vi "Act_cmd (SubVI).vi"(4 "W_b [rad/s]":dbl[](array[numeric]), 6 "Angles [rad]":dbl[](array[numeric]), 8 "TVA_old [rad]":dbl[](array[numeric]), 11 "TVA_cmd [rad]":dbl[](array[numeric])) -> (1 "roll1":dbl, 2 "Act315_Act225":dbl[](array[numeric]))   [LabVIEW 2011]
panel:
  out "TVA_control_time [s]":dbl
  in  "T [s]":dbl=0.06 format="%#_13g"
  out "roll_angle [rad]":dbl
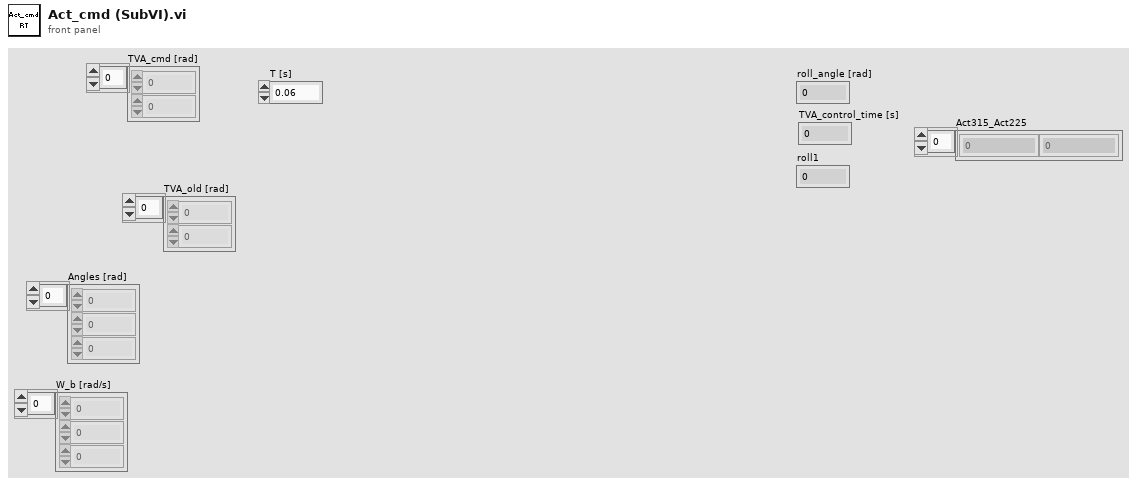
[diagram p1: front panel]
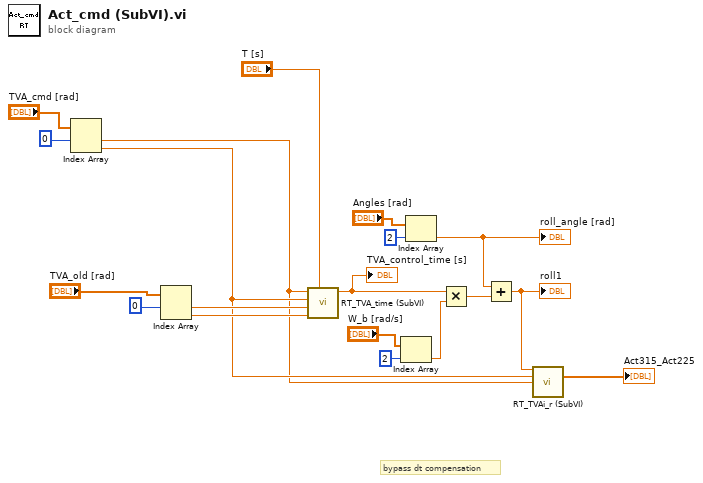
[diagram p0: block diagram]
diagram:
  # "bypass dt compensation"
  n1 = Index Array(array="TVA_cmd [rad]", index #1=0 ("disabled index (col)")) -> (element #1=w4:dbl, element #2=w5:dbl)  [unwired: 1 in]
  n2 = Index Array(array="TVA_old [rad]", index #1=0 ("disabled index (col)")) -> (element #1=w15:dbl, element #2=w14:dbl)  [unwired: 1 in]
  n3 = call "RT_TVA_time (SubVI).vi"("T [s]"="T [s]", "TVA_y_old"=w14, "TVA_p_old"=w15, "TVA_y"=w5, "TVA_p"=w4) -> ("TVA_control_time [s]"=w3:dbl)  [unwired: 6 in]
  "TVA_control_time [s]" <- w3
  n4 = Index Array(array="W_b [rad/s]", index=2) -> (element=w7:dbl)
  n5 = Index Array(array="Angles [rad]", index=2) -> (element=w2:dbl)
  "roll_angle [rad]" <- w2
  n6 = Multiply(x=w3, y=w7) -> (x*y=w8:dbl)
  n7 = Add(x=w2, y=w8) -> (x+y=w1:dbl)
  "roll1" <- w1
  n8 = call "RT_TVAi_r (SubVI).vi"("roll1"=w1, "TVA_p"=w5, "TVA_y"=w4) -> ("Act315_Act225"=→"Act315_Act225":dbl[])  [unwired: 12 in]
